vi "Generate Month Load SQL Query.vi"(8 "error in (no error)":errorcluster, 10 "Year-Mo":string, 11 "Banking Statement in":refnum<class "Banking Transactions.lvclass">) -> (0 "error out":errorcluster, 2 "SQL Query":string, 3 "Banking Statement out":refnum<class "Banking Transactions.lvclass">)   [LabVIEW 2018, in "Banking Transactions.lvclass"]
uses:
  Banking Transactions.lvclass
  Statement/TransactionList.lvclass
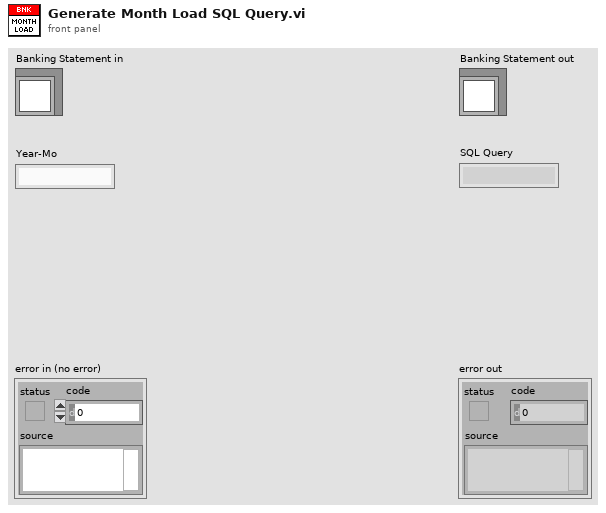
[diagram p1: front panel]
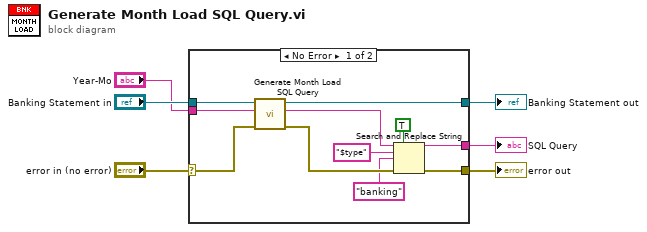
[diagram p0: block diagram]
diagram:
  n1 = case shown="No Error" "error in (no error)" {
    selector: "error in (no error)" -> [w10 w19]
    tunnel: "Banking Statement in" -> [w17 w18]
    tunnel: [w12 w19] -> w3
    tunnel: [w11 _] -> w2
    tunnel: "Year-Mo" -> [w9 _]
    tunnel: [w8 w18] -> w1
    frame No Error {
      n2 = call-parent "Generate Month Load SQL Query.vi"("error in (no error)"=w10, "Year-Mo"=w9, "Statement in"=w17) -> ("error out"=w15:errorcluster, "SQL Query"=w16:string, "Statement out"=w8:refnum<class "Banking Transactions.lvclass">)  [unwired: 6 in]
      n3 = Search and Replace String(replace all?=TRUE ("replace all? (F)"), input string=w16, search string="$type", replace string="banking", error in=w15) -> (result string=w11:string, error out=w12:errorcluster)  [unwired: 3 in, 2 out]
    }
    frame Error {
    }
  }
  "error out" <- w3
  "Banking Statement out" <- w1
  "SQL Query" <- w2
